vi "Demo.vi"() -> ()   [LabVIEW 2018]
uses:
  <vilib>/vision/Image Controls.llb/IMAQ Image.ctl
  VsyCam.dll
panel:
  out "ImageData":T1
  out "Image":T1(plugin-control)
  out "版本号":dbl
  in  "同步切换":bool
  in  "保存":bool
  out "采集状态":string
  out "曝光时间":dbl
  in  "曝光设置(us)":i32(c297)
  out "帧率":dbl
  in  "帧率设置(fps)":i32(c297)
  out "偏置":dbl
  in  "偏置设置":i32(c297)
  out "增益":dbl
  in  "增益设置(dB)":i32(c297)
  out "采集套接字":i32
  out "控制套接字":i32
  out "采集帧数":i32
  out "心跳返回值":i32
  out "连接状态":bool
  in  "建立连接":bool
  out "相机IP":string[](array[string])
  in  "搜寻相机":bool
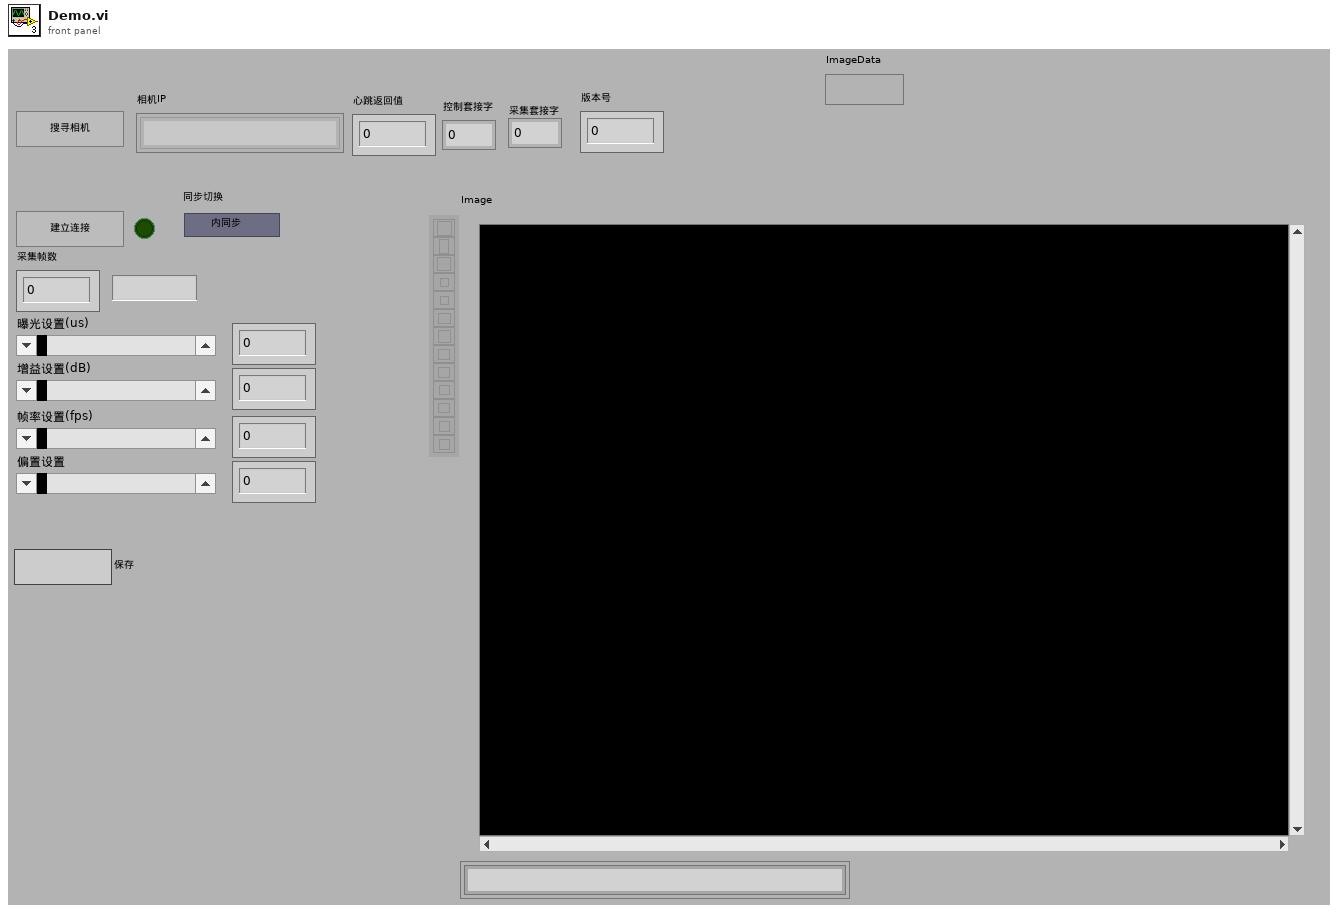
[diagram p1: front panel]
types:
  T1 = typedef "IMAQ Image.ctl" = refnum<image>
  T2 = typedef "Image Type" = u32
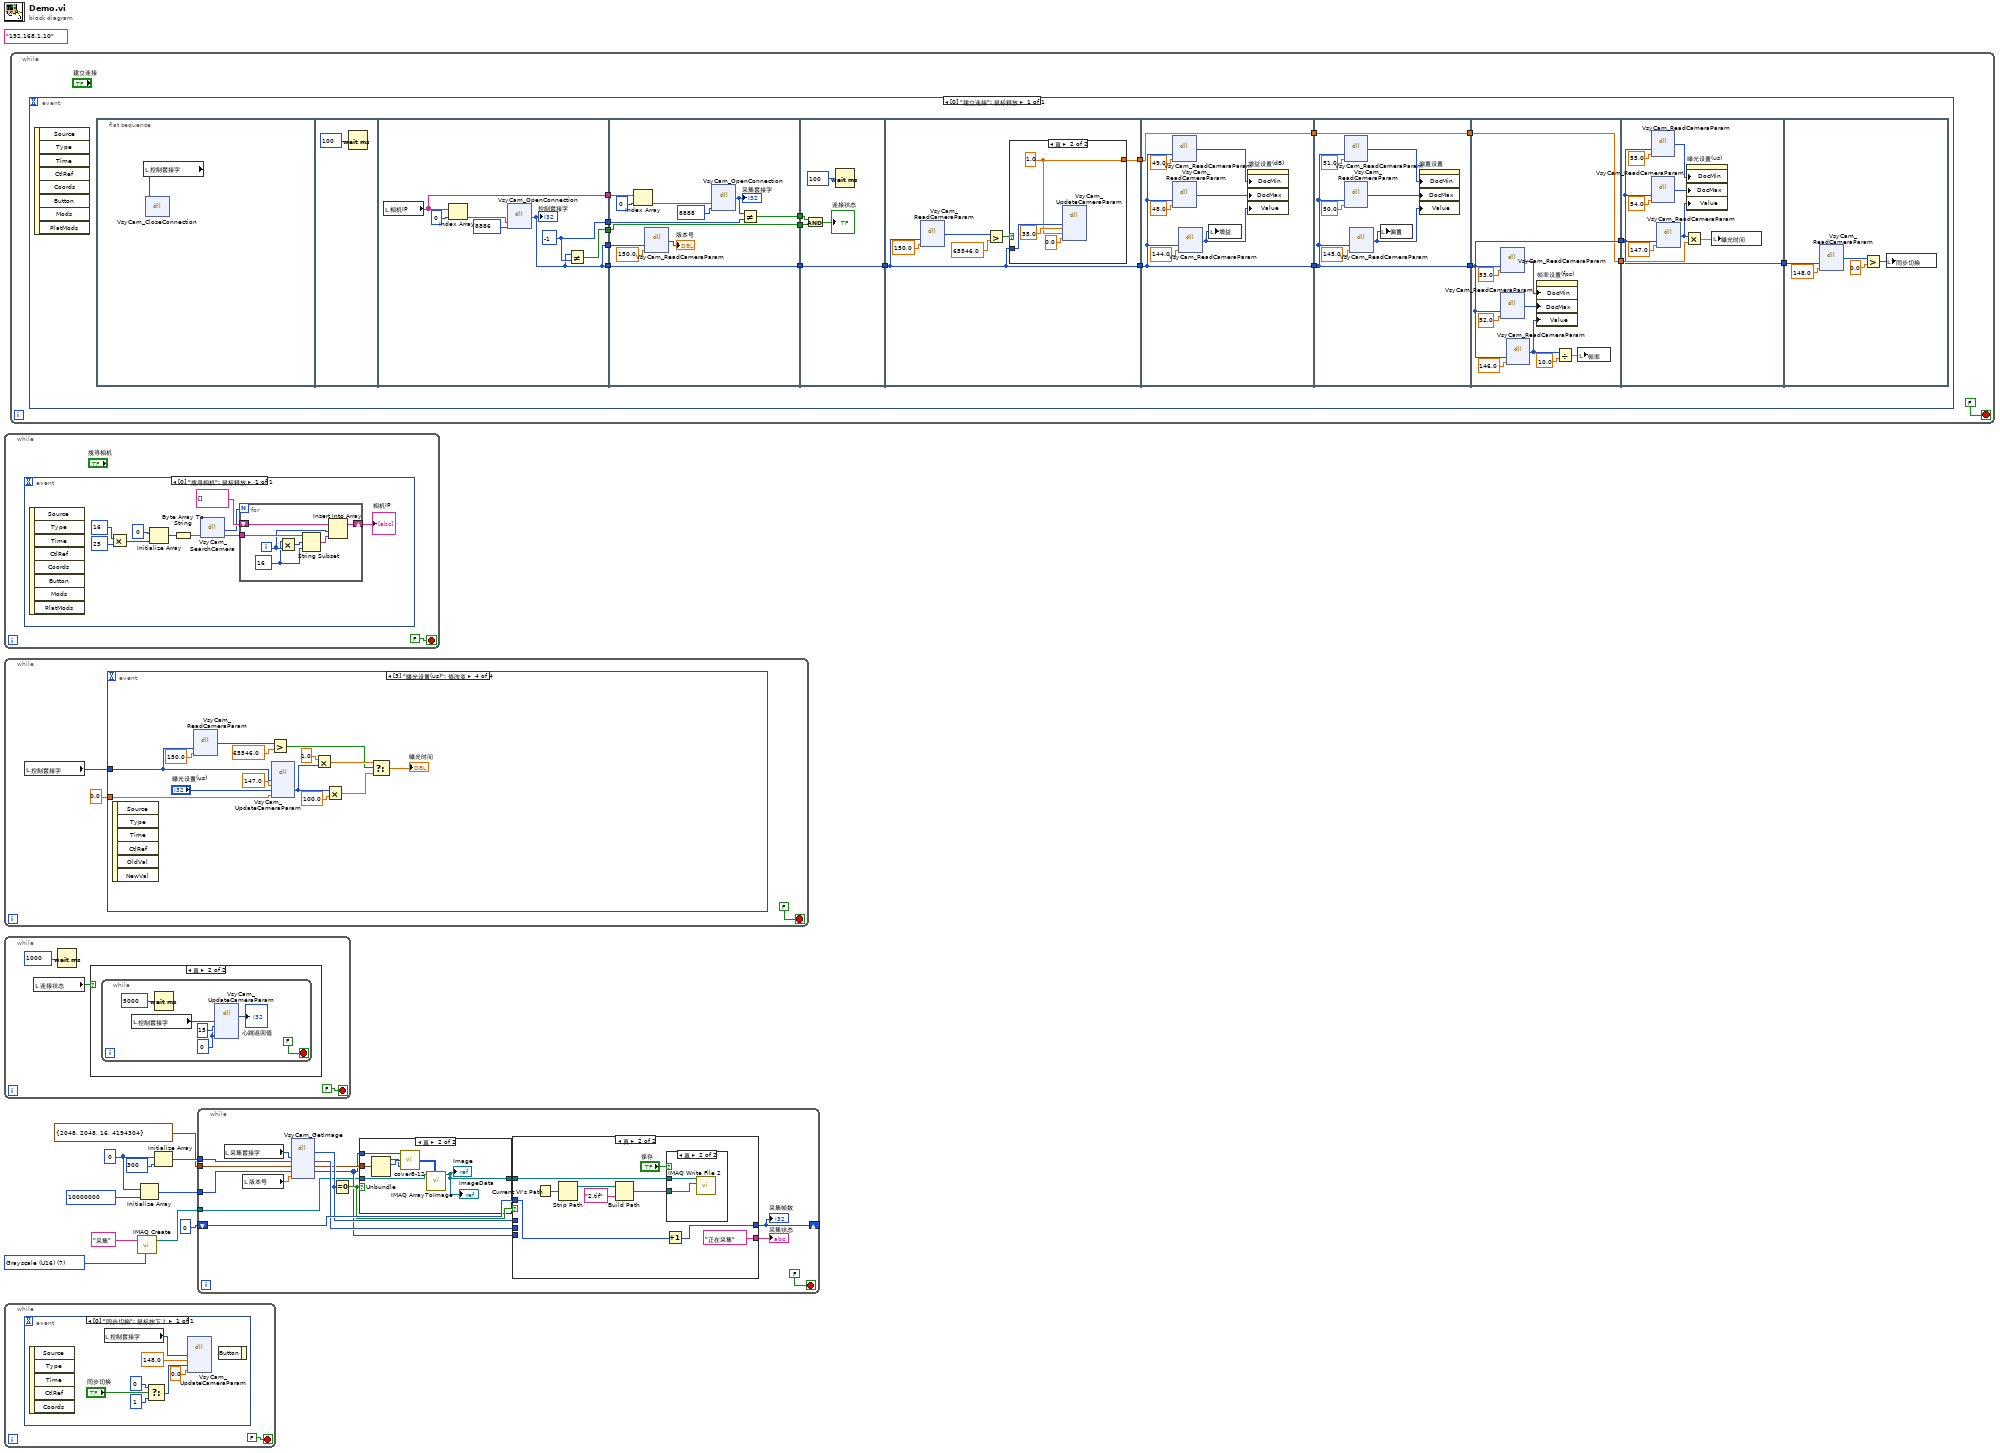
[diagram p0: block diagram]
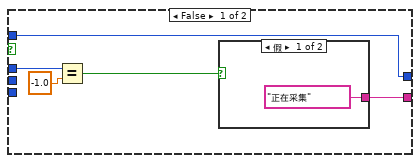
[diagram p3: hidden frame]
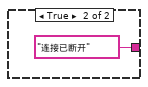
[diagram p4: hidden frame]
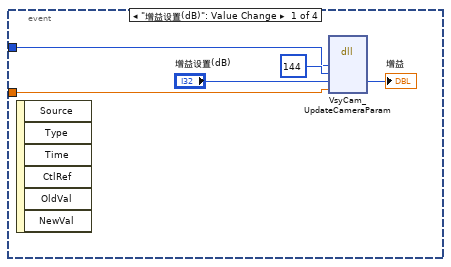
[diagram p6: hidden frame]
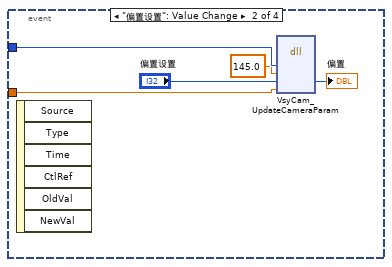
[diagram p7: hidden frame]
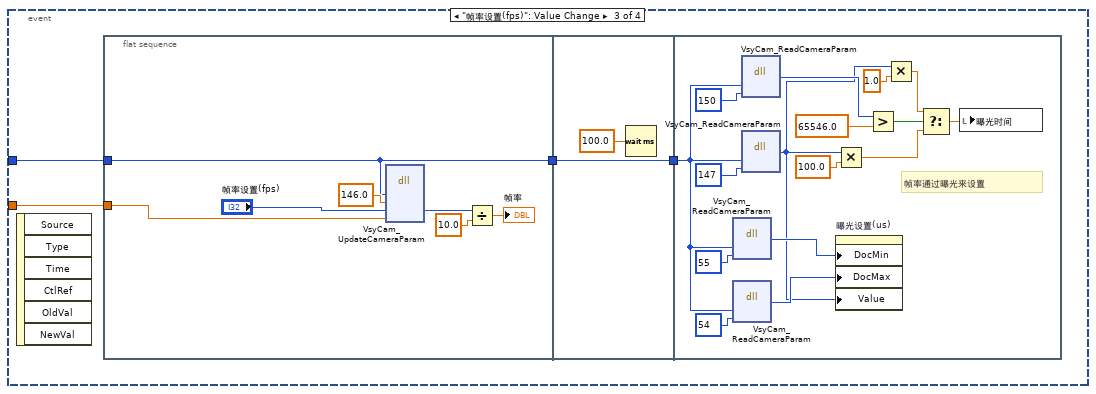
[diagram p8: hidden frame]
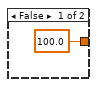
[diagram p10: hidden frame]
diagram:
  w1 = T2 7 items=["Grayscale (U8)", "Grayscale (I16)", "Grayscale (SGL)", "Complex (CSG)", "RGB (U32)", "HSL (U32)", "RGB (U64)", "Grayscale (U16)"] ("Image Type")
  (unwired) "192.168.1.10" ("元素")
  w6 = u8 0
  n1 = while {
    stop <- FALSE stop-if-true
    n2 = event shown="[0] \"搜寻相机\": 鼠标释放" {
      selector: _ -> [_]
      dyn-events: _ -> [_]
      timeout: _ -> [_]
      event "搜寻相机": Mouse Up {
        n3 = event-data() -> ()  [unwired: 1 in, 8 out]
        n4 = Multiply(x=16, y=25) -> (x*y=w14:i32)
        n5 = Initialize Array(0, w14) -> (w13:i32[])
        n6 = Byte Array To String(unsigned byte array=w13) -> (string=w12:string)
        n7 = dll-call lib="PTH2?abs D做的项目航天测量软件相机\nVsyCam.dll" fn="VsyCam_SearchCamera"("ipArray"=w12) -> ("返回类型"=w19:i32, "ipArray"=w18:string)  [unwired: 3 in, 2 out]
        n8 = for {
          N: w19 -> [_]
          tunnel: w18 -> [w28]
          shift-right: [w26] -> w21
          shift-left: string[] [] ("相机IP") -> [w27]
          i -> [w24]
          w22 = 16
          n9 = Multiply(x=w22, y=w24) -> (x*y=w23:i32)
          n10 = String Subset(string=w28, offset (0)=w23, length (rest)=w22) -> (substring=w25:string)
          n11 = Insert Into Array(array=w27, index=w24, new element=w25) -> (w26:string[])
        }
        "相机IP" <- w21
      }
    }
  }
  n12 = while {
    stop <- FALSE stop-if-true
    n13 = local read "控制套接字"() -> (w29:i32)
    n14 = event shown="[3] \"曝光设置(us)\": 值改变" {
      selector: _ -> [_ _ _ _]
      dyn-events: _ -> [_ _ _ _]
      timeout: _ -> [_ _ _ _]
      tunnel: 0.0 -> [w33 w41 w45 w83]
      tunnel: w29 -> [w32 w40 w44 w74]
      event "增益设置(dB)": Value Change {
        n15 = event-data() -> ()  [unwired: 1 in, 6 out]
        n16 = dll-call lib="PTH2?abs D做的项目航天测量软件相机\nVsyCam.dll" fn="VsyCam_UpdateCameraParam"("sockFd"=w32, "command"=144, "value"="增益设置(dB)", "ack"=w33) -> ("value"=→"增益":i32)  [unwired: 7 in, 2 out]
      }
      event "偏置设置": Value Change {
        n17 = event-data() -> ()  [unwired: 1 in, 6 out]
        n18 = dll-call lib="PTH2?abs D做的项目航天测量软件相机\nVsyCam.dll" fn="VsyCam_UpdateCameraParam"("sockFd"=w40, "command"=145.0, "value"="偏置设置", "ack"=w41) -> ("value"=→"偏置":i32)  [unwired: 7 in, 2 out]
      }
      event "帧率设置(fps)": Value Change {
        n19 = event-data() -> ()  [unwired: 1 in, 6 out]
        n20 = flat-sequence {
          tunnel: w45 -> [w52]
          tunnel: w44 -> [w46]
          tunnel: [w46] -> w43
          tunnel: w43 -> [w54]
          tunnel: [w54] -> w42
          tunnel: w42 -> [w63]
          frame #0 {
            n21 = dll-call lib="PTH2?abs D做的项目航天测量软件相机\nVsyCam.dll" fn="VsyCam_UpdateCameraParam"("sockFd"=w46, "command"=146.0, "value"="帧率设置(fps)", "ack"=w52) -> ("value"=w49:i32)  [unwired: 7 in, 2 out]
            n22 = Divide(x=w49, y=10.0) -> (x/y=→"帧率":dbl)
          }
          frame #1 {
            n23 = Wait (ms)(milliseconds to wait=100.0) -> ()  [unwired: 1 out]
          }
          frame #2 {
            # "帧率通过曝光来设置"
            n24 = dll-call lib="PTH2?abs D做的项目航天测量软件相机\nVsyCam.dll" fn="VsyCam_ReadCameraParam"("sockFd"=w63, "cmd"=55) -> ("返回类型"=w70:i32)  [unwired: 5 in, 2 out]
            n25 = dll-call lib="PTH2?abs D做的项目航天测量软件相机\nVsyCam.dll" fn="VsyCam_ReadCameraParam"("sockFd"=w63, "cmd"=54) -> ("返回类型"=w69:i32)  [unwired: 5 in, 2 out]
            n26 = dll-call lib="PTH2?abs D做的项目航天测量软件相机\nVsyCam.dll" fn="VsyCam_ReadCameraParam"("sockFd"=w63, "cmd"=150) -> ("返回类型"=w62:i32)  [unwired: 5 in, 2 out]
            n27 = dll-call lib="PTH2?abs D做的项目航天测量软件相机\nVsyCam.dll" fn="VsyCam_ReadCameraParam"("sockFd"=w63, "cmd"=147) -> ("返回类型"=w56:i32)  [unwired: 5 in, 2 out]
            n28 = Multiply(x=w56, y=100.0) -> (x*y=w55:dbl)
            n29 = property on="曝光设置(us)" class="Scroll (严格)"("DocMin"=w70, "DocMax"=w69, "Value"=w56) -> ()  [unwired: 2 in, 2 out]
            n30 = Greater?(x=w62, y=65546.0) -> (0:w61:bool)
            n31 = Multiply(x=w56, y=1.0) -> (x*y=w59:dbl)
            n32 = Select(t=w59, s=w61, f=w55) -> (s? t:f=w58:dbl)
            n33 = local write "曝光时间"(w58) -> ()
          }
        }
      }
      event "曝光设置(us)": Value Change {
        n34 = event-data() -> ()  [unwired: 1 in, 6 out]
        n35 = dll-call lib="PTH2?abs D做的项目航天测量软件相机\nVsyCam.dll" fn="VsyCam_ReadCameraParam"("sockFd"=w74, "cmd"=150.0) -> ("返回类型"=w72:i32)  [unwired: 5 in, 2 out]
        n36 = Greater?(x=w72, y=65546.0) -> (0:w71:bool)
        n37 = dll-call lib="PTH2?abs D做的项目航天测量软件相机\nVsyCam.dll" fn="VsyCam_UpdateCameraParam"("sockFd"=w74, "command"=147.0, "value"="曝光设置(us)", "ack"=w83) -> ("value"=w79:i32)  [unwired: 7 in, 2 out]
        n38 = Multiply(x=1.0, y=w79) -> (x*y=w78:dbl)
        n39 = Multiply(x=w79, y=100.0) -> (x*y=w77:dbl)
        n40 = Select(t=w78, s=w71, f=w77) -> (s? t:f=→"曝光时间":dbl)
      }
    }
  }
  n41 = while {
    stop <- FALSE stop-if-true
    n42 = local read "连接状态"() -> (w86:bool)
    n43 = Wait (ms)(milliseconds to wait=u32 1000 ("等待时间（毫秒）")) -> ()  [unwired: 1 out]
    n44 = case shown="真" w86 {
      frame False {
      }
      frame True {
        n45 = while {
          stop <- FALSE stop-if-true
          w90 = 0
          n46 = local read "控制套接字"() -> (w88:i32)
          n47 = Wait (ms)(milliseconds to wait=5000) -> ()  [unwired: 1 out]
          n48 = dll-call lib="PTH2?abs D做的项目航天测量软件相机\nVsyCam.dll" fn="VsyCam_UpdateCameraParam"("sockFd"=w88, "command"=15, "value"=w90, "ack"=w90) -> ("返回类型"=→"心跳返回值":i32)  [unwired: 7 in, 2 out]
        }
      }
    }
  }
  n49 = while {
    stop <- FALSE stop-if-true
    n50 = event shown="[0] \"同步切换\": 鼠标按下？" {
      selector: _ -> [_]
      dyn-events: _ -> [_]
      timeout: _ -> [_]
      event "同步切换": Mouse Down? {
        n51 = event-data() -> ()  [unwired: 1 in, 5 out]
        n52 = local read "控制套接字"() -> (w101:i32)
        n53 = Select(t=0, s="同步切换", f=1) -> (s? t:f=w98:i32)
        n54 = dll-call lib="PTH2?abs D做的项目航天测量软件相机\nVsyCam.dll" fn="VsyCam_UpdateCameraParam"("sockFd"=w101, "command"=148.0, "value"=w98, "ack"=0.0) -> ()  [unwired: 8 in, 2 out]
        n55 = event-data() -> ()  [unwired: 2 in, 1 out]
      }
    }
  }
  n56 = while {
    stop <- FALSE stop-if-true
    n57 = event shown="[0] \"建立连接\": 鼠标释放" {
      selector: _ -> [_]
      dyn-events: _ -> [_]
      timeout: _ -> [_]
      event "建立连接": Mouse Up {
        n58 = event-data() -> ()  [unwired: 1 in, 8 out]
        n59 = flat-sequence {
          tunnel: [w127] -> w120
          tunnel: [w125] -> w119
          tunnel: [w124] -> w117
          tunnel: [w123] -> w114
          tunnel: [w123] -> w104
          tunnel: w120 -> [w140]
          tunnel: w119 -> [w137]
          tunnel: [w136] -> w118
          tunnel: w117 -> [w136]
          tunnel: [w135] -> w116
          tunnel: [w134] -> w115
          tunnel: w114 -> [w134]
          tunnel: w104 -> [w132]
          tunnel: w118 -> [w146]
          tunnel: w116 -> [w145]
          tunnel: w115 -> [w143]
          tunnel: [w143] -> w110
          tunnel: w110 -> [w150]
          tunnel: [w150] -> w109
          tunnel: [w149] -> w108
          tunnel: w109 -> [w159]
          tunnel: [w159] -> w113
          tunnel: w108 -> [w158]
          tunnel: [w158] -> w107
          tunnel: w113 -> [w167]
          tunnel: [w167] -> w112
          tunnel: w107 -> [w166]
          tunnel: [w166] -> w106
          tunnel: w112 -> [w175]
          tunnel: [w175] -> w111
          tunnel: w106 -> [w174]
          tunnel: [w174] -> w105
          tunnel: w111 -> [w184]
          tunnel: w105 -> [w187]
          tunnel: [w184] -> w103
          tunnel: w103 -> [w197]
          frame #0 {
            n60 = local read "控制套接字"() -> (w121:i32)
            n61 = dll-call lib="PTH2?abs D做的项目航天测量软件相机\nVsyCam.dll" fn="VsyCam_CloseConnection"("sockFd"=w121) -> ()  [unwired: 5 in, 2 out]
          }
          frame #1 {
            n62 = Wait (ms)(milliseconds to wait=u32 100 ("等待时间（毫秒）")) -> ()  [unwired: 1 out]
          }
          frame #2 {
            w125 = -1
            n63 = local read "相机IP"() -> (w127:string[])
            n64 = Index Array(array=w127, index=0) -> (element=w128:string)
            n65 = dll-call lib="PTH2?abs D做的项目航天测量软件相机\nVsyCam.dll" fn="VsyCam_OpenConnection"("ip"=w128, "port"=8886) -> ("返回类型"=w123:i32)  [unwired: 5 in, 2 out]
            "控制套接字" <- w123
            n66 = Not Equal?(x=w123, y=w125) -> (x != y?=w124:bool)
          }
          frame #3 {
            n67 = Index Array(array=w140, index=0) -> (element=w141:string)
            n68 = dll-call lib="PTH2?abs D做的项目航天测量软件相机\nVsyCam.dll" fn="VsyCam_ReadCameraParam"("sockFd"=w132, "cmd"=150.0) -> ("返回类型"=→"版本号":i32)  [unwired: 5 in, 2 out]
            n69 = dll-call lib="PTH2?abs D做的项目航天测量软件相机\nVsyCam.dll" fn="VsyCam_OpenConnection"("ip"=w141, "port"=8888) -> ("返回类型"=w133:i32)  [unwired: 5 in, 2 out]
            "采集套接字" <- w133
            n70 = Not Equal?(x=w133, y=w137) -> (x != y?=w135:bool)
          }
          frame #4 {
            n71 = And(x=w145, y=w146) -> (x .and. y?=→"连接状态":bool)
            n72 = Wait (ms)(milliseconds to wait=u32 100 ("等待时间（毫秒）")) -> ()  [unwired: 1 out]
          }
          frame #5 {
            n73 = dll-call lib="PTH2?abs D做的项目航天测量软件相机\nVsyCam.dll" fn="VsyCam_ReadCameraParam"("sockFd"=w150, "cmd"=150.0) -> ("返回类型"=w147:i32)  [unwired: 5 in, 2 out]
            n74 = Greater?(x=w147, y=65546.0) -> (0:w148:bool)
            n75 = case shown="真" w148 {
              tunnel: w150 -> [_ w157]
              tunnel: [100.0 w154] -> w149
              frame False {
              }
              frame True {
                w154 = 1.0
                n76 = dll-call lib="PTH2?abs D做的项目航天测量软件相机\nVsyCam.dll" fn="VsyCam_UpdateCameraParam"("sockFd"=w157, "command"=35.0, "value"=w154, "ack"=0.0) -> ()  [unwired: 8 in, 2 out]
              }
            }
          }
          frame #6 {
            n77 = dll-call lib="PTH2?abs D做的项目航天测量软件相机\nVsyCam.dll" fn="VsyCam_ReadCameraParam"("sockFd"=w159, "cmd"=49.0) -> ("返回类型"=w164:i32)  [unwired: 5 in, 2 out]
            n78 = dll-call lib="PTH2?abs D做的项目航天测量软件相机\nVsyCam.dll" fn="VsyCam_ReadCameraParam"("sockFd"=w159, "cmd"=48.0) -> ("返回类型"=w165:i32)  [unwired: 5 in, 2 out]
            n79 = dll-call lib="PTH2?abs D做的项目航天测量软件相机\nVsyCam.dll" fn="VsyCam_ReadCameraParam"("sockFd"=w159, "cmd"=144.0) -> ("返回类型"=w160:i32)  [unwired: 5 in, 2 out]
            n80 = local write "增益"(w160) -> ()
            n81 = property on="增益设置(dB)" class="Scroll (严格)"("DocMin"=w164, "DocMax"=w165, "Value"=w160) -> ()  [unwired: 2 in, 2 out]
          }
          frame #7 {
            n82 = dll-call lib="PTH2?abs D做的项目航天测量软件相机\nVsyCam.dll" fn="VsyCam_ReadCameraParam"("sockFd"=w167, "cmd"=51.0) -> ("返回类型"=w171:i32)  [unwired: 5 in, 2 out]
            n83 = dll-call lib="PTH2?abs D做的项目航天测量软件相机\nVsyCam.dll" fn="VsyCam_ReadCameraParam"("sockFd"=w167, "cmd"=50.0) -> ("返回类型"=w172:i32)  [unwired: 5 in, 2 out]
            n84 = dll-call lib="PTH2?abs D做的项目航天测量软件相机\nVsyCam.dll" fn="VsyCam_ReadCameraParam"("sockFd"=w167, "cmd"=145.0) -> ("返回类型"=w173:i32)  [unwired: 5 in, 2 out]
            n85 = local write "偏置"(w173) -> ()
            n86 = property on="偏置设置" class="Scroll (严格)"("DocMin"=w171, "DocMax"=w172, "Value"=w173) -> ()  [unwired: 2 in, 2 out]
          }
          frame #8 {
            n87 = dll-call lib="PTH2?abs D做的项目航天测量软件相机\nVsyCam.dll" fn="VsyCam_ReadCameraParam"("sockFd"=w175, "cmd"=53.0) -> ("返回类型"=w183:i32)  [unwired: 5 in, 2 out]
            n88 = dll-call lib="PTH2?abs D做的项目航天测量软件相机\nVsyCam.dll" fn="VsyCam_ReadCameraParam"("sockFd"=w175, "cmd"=52.0) -> ("返回类型"=w182:i32)  [unwired: 5 in, 2 out]
            n89 = dll-call lib="PTH2?abs D做的项目航天测量软件相机\nVsyCam.dll" fn="VsyCam_ReadCameraParam"("sockFd"=w175, "cmd"=146.0) -> ("返回类型"=w178:i32)  [unwired: 5 in, 2 out]
            n90 = property on="帧率设置(fps)" class="Scroll (严格)"("DocMin"=w183, "DocMax"=w182, "Value"=w178) -> ()  [unwired: 2 in, 2 out]
            n91 = Divide(x=w178, y=10.0) -> (x/y=w177:dbl)
            n92 = local write "帧率"(w177) -> ()
          }
          frame #9 {
            n93 = dll-call lib="PTH2?abs D做的项目航天测量软件相机\nVsyCam.dll" fn="VsyCam_ReadCameraParam"("sockFd"=w184, "cmd"=55.0) -> ("返回类型"=w186:i32)  [unwired: 5 in, 2 out]
            n94 = dll-call lib="PTH2?abs D做的项目航天测量软件相机\nVsyCam.dll" fn="VsyCam_ReadCameraParam"("sockFd"=w184, "cmd"=54.0) -> ("返回类型"=w185:i32)  [unwired: 5 in, 2 out]
            n95 = dll-call lib="PTH2?abs D做的项目航天测量软件相机\nVsyCam.dll" fn="VsyCam_ReadCameraParam"("sockFd"=w184, "cmd"=147.0) -> ("返回类型"=w188:i32)  [unwired: 5 in, 2 out]
            n96 = Multiply(x=w188, y=w187) -> (x*y=w189:dbl)
            n97 = property on="曝光设置(us)" class="Scroll (严格)"("DocMin"=w186, "DocMax"=w185, "Value"=w188) -> ()  [unwired: 2 in, 2 out]
            n98 = local write "曝光时间"(w189) -> ()
          }
          frame #10 {
            n99 = dll-call lib="PTH2?abs D做的项目航天测量软件相机\nVsyCam.dll" fn="VsyCam_ReadCameraParam"("sockFd"=w197, "cmd"=148.0) -> ("返回类型"=w194:i32)  [unwired: 5 in, 2 out]
            n100 = Greater?(x=w194, y=0.0) -> (0:w193:bool)
            n101 = local write "同步切换"(w193) -> ()
          }
        }
      }
    }
  }
  n102 = call "IMAQ Create"("Image Name"="采集", "Image Type"=w1) -> ("New Image"=w2:T1)  [unwired: 3 in, 1 out]
  n103 = Initialize Array(w6, 10000000) -> (w8:u8[])
  n104 = Initialize Array(w6, 300) -> (w9:u8[])
  n105 = while {
    tunnel: w9 -> [w213]
    tunnel: w8 -> [w212]
    shift-right: [w207] -> _
    shift-left: 0 -> [w209]
    tunnel: cluster{i32, i32, i32, i32} {2048, 2048, 16, 4194304} ("簇") -> [w202]
    tunnel: w2 -> [w199]
    stop <- FALSE stop-if-true
    n106 = local read "采集套接字"() -> (w211:i32)
    n107 = local read "版本号"() -> (w205:dbl)
    n108 = dll-call lib="PTH2?abs D做的项目航天测量软件相机\nVsyCam.dll" fn="VsyCam_GetImage"("sockFd"=w211, "Header"=w213, "ImgInfo"=w202, "Data"=w212, "version"=w205) -> ("返回类型"=w206:i32, "Header"=w204:u8[], "ImgInfo"=w201:cluster{i32, i32, i32, i32}, "Data"=w200:u8[])  [unwired: 5 in, 2 out]
    n109 = Equal To 0?(x=w206) -> (x = 0?=w203:bool)
    n110 = case shown="真" w203 {
      tunnel: w201 -> [_ w217]
      tunnel: w200 -> [_ w219]
      tunnel: w199 -> [w214 w221]
      tunnel: [w214 w220] -> w198
      frame False {
      }
      frame True {
        n111 = Unbundle(w217) -> (w215:i32, w216:i32)  [unwired: 2 out]
        n112 = call "cover8-12.vi"("H"=w215, "W"=w216, "Image Data"=w219) -> ("PIC Out"=w218:u16[][])
        n113 = call "IMAQ ArrayToImage"("Image Pixels (U16)"=w218, "Image"=w221) -> ("Image Out"=w220:T1)  [unwired: 8 in, 1 out]
        "Image" <- w220
        "ImageData" <- w220
      }
    }
    n114 = case shown="真" w203 {
      tunnel: w200 -> [_ _]
      tunnel: w204 -> [_ _]
      tunnel: w209 -> [w225 w235]
      tunnel: [w226 "正在采集"] -> w208
      tunnel: [w225 w236] -> w207
      tunnel: w206 -> [w222 _]
      tunnel: w198 -> [_ w233]
      frame False {
        n115 = Equal?(x=w222, y=-1.0) -> (x = y?=w223:bool)
        n116 = case shown="假" w223 {
          tunnel: ["正在采集" "连接已断开"] -> w226
          frame False {
          }
          frame True {
          }
        }
      }
      frame True {
        n117 = Current VI's Path() -> (path=w232:path)
        n118 = Strip Path(path=w232) -> (stripped path=w231:path)  [unwired: 1 out]
        n119 = Build Path(base path=w231, name or relative path="2.tif" ("名称或相对路径")) -> (appended path=w229:path)
        n120 = Increment(x=w235) -> (x+1=w236:i32)
        n121 = case shown="真" "保存" {
          tunnel: w233 -> [_ w239]
          tunnel: w229 -> [_ w238]
          frame False {
          }
          frame True {
            n122 = call-poly "IMAQ Write File 2"("File Path"=w238, "Image"=w239) -> ()  [unwired: 8 in, 2 out]
          }
        }
      }
    }
    "采集状态" <- w208
    "采集帧数" <- w207
  }
